vi "System Explorer - Copy Templates for System Explorer.vi"(8 "error in (no error)":errorcluster, 11 "System Explorer folder":path) -> (0 "error out":errorcluster)   [LabVIEW 2015]
doc: "Copy the templates for the System Explorer library into the System Explorer folder and disconnect the templates from the owning library."
uses:
  Constants/Constants TypDef/CD System Explorer lvlib.ctl
  Constants/CD System Explorer lvlib.vi
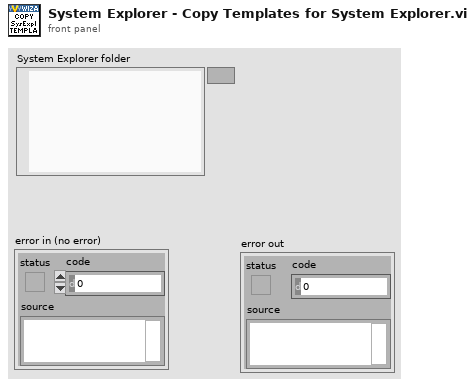
[diagram p1: front panel]
types:
  T1 = typedef "CD System Explorer lvlib.ctl" = enum16{"LibraryFileName", "LibraryFolderName", "System Explorer.FolderName", "System Explorer.Dynamically Called.FolderName", "System Explorer.Dynamically Called.Extra Pages.FolderName", "System Explorer.Dynamically Called.Extra Pages.TemplatePathAndName", "System Explorer.Dynamically Called.Main Page.VIName", "System Explorer.Dynamically Called.Main Page.TemplatePathAndName", "System Explorer.Dynamically Called.Initialization VI.VIName", "System Explorer.Dynamically Called.Initialization VI.TemplatePathAndName", "System Explorer.SubVI.FolderName", "System Explorer.Types.FolderName"}
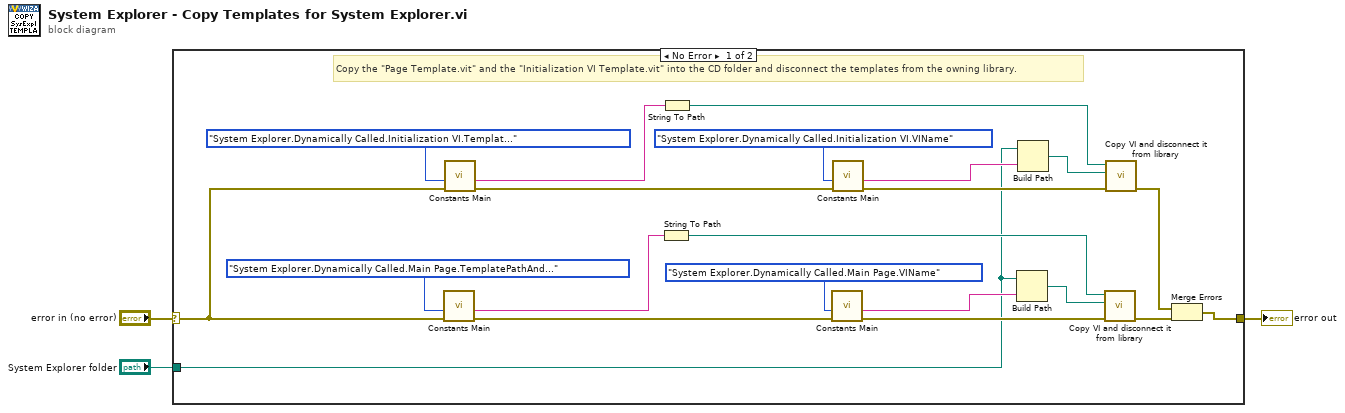
[diagram p0: block diagram]
diagram:
  n1 = case shown="No Error" "error in (no error)" {
    selector: "error in (no error)" -> [w8 w25]
    tunnel: "System Explorer folder" -> [w7 _]
    tunnel: [w4 w25] -> w1
    frame No Error {
      # "Copy the \"Page Template.vit\" and the \"Initialization VI Template.vit\" into the CD folder and disconnect the templates from the owning library."
      n2 = call-poly "Constants Main.vi"("error in (no error)"=w8, "Action"=CD_System_Explorer_lvlib."System Explorer.Dynamically Called.Main Page.TemplatePathAndName") -> ("error out"=w17:errorcluster, "Output"=w20:string)  [unwired: 8 in]
      n3 = call-poly "Constants Main.vi"("error in (no error)"=w8, "Action"=CD_System_Explorer_lvlib."System Explorer.Dynamically Called.Initialization VI.TemplatePathAndName") -> ("error out"=w16:errorcluster, "Output"=w13:string)  [unwired: 8 in]
      n4 = String To Path(string=w20) -> (path=w18:path)
      n5 = String To Path(string=w13) -> (path=w15:path)
      n6 = call-poly "Constants Main.vi"("error in (no error)"=w17, "Action"=CD_System_Explorer_lvlib."System Explorer.Dynamically Called.Main Page.VIName") -> ("error out"=w23:errorcluster, "Output"=w22:string)  [unwired: 8 in]
      n7 = call-poly "Constants Main.vi"("error in (no error)"=w16, "Action"=CD_System_Explorer_lvlib."System Explorer.Dynamically Called.Initialization VI.VIName") -> ("error out"=w10:errorcluster, "Output"=w11:string)  [unwired: 8 in]
      n8 = Build Path(base path=w7, name or relative path=w22) -> (appended path=w24:path)
      n9 = Build Path(base path=w7, name or relative path=w11) -> (appended path=w9:path)
      n10 = call "Copy VI and disconnect it from library.vi"("error in (no error)"=w23, "VI Target Path"=w24, "VI Source Path"=w18) -> ("error out"=w5:errorcluster)  [unwired: 8 in]
      n11 = call "Copy VI and disconnect it from library.vi"("error in (no error)"=w10, "VI Target Path"=w9, "VI Source Path"=w15) -> ("error out"=w6:errorcluster)  [unwired: 8 in]
      n12 = Merge Errors(w6, w5) -> (w4:errorcluster)
    }
    frame Error {
    }
  }
  "error out" <- w1
